vi "Path_Test_TankRobot_ScanIndex_CreateFile.vi"() -> ()   [LabVIEW 2018]
uses:
  Pathfinder-Lib/VIs/Waypoint.ctl
  <vilib>/Rock Robotics/WPI/DriverStation/WPI_DriverStationRobotMode2.ctl
  Pathfinder-Lib/VIs/Wheel_Ctrl_Path_Element.ctl
  Pathfinder-Lib/VIs/Wheel_Ctrl_Path.ctl
  Pathfinder-Lib/Pathfinder.lvlib
  Robot Global Data.vi
  <vilib>/Rock Robotics/SystemInterfaces/AI/FPGA_AIGyroChannel.ctl
  <vilib>/Rock Robotics/Network Tables/NT Write Number.vi
  <vilib>/Rock Robotics/WPI/Counter/WPI_CounterDigitalInputToDigitalSource.vi
  <vilib>/Rock Robotics/SystemInterfaces/DIO/FPGA_DIOChannel.ctl
  <vilib>/Rock Robotics/WPI/Encoder/WPI_EncoderType.ctl
  <vilib>/Rock Robotics/Network Tables/NT Write Numeric Array.vi
  <vilib>/addons/control/pid/NI_PID_pid.lvlib
  <vilib>/Rock Robotics/SystemInterfaces/DIO/FPGA_DIOPWMChannel.ctl
  <vilib>/Rock Robotics/WPI/SafetyOutput/WPI_SafetyOutputConfigMenu.ctl
  Secret_Control_Library_Protected/Secret_Control_Library_Protected.lvlib
  <vilib>/addons/control/pid/pid.llb/PID (DBL).vi
  <vilib>/Rock Robotics/WPI/Gyro/WPI_GyroAnalogOpen.vi
  <vilib>/Rock Robotics/WPI/RobotDrive/WPI_RobotDriveOpen2MotorWithTalon.vi
panel:
  out "Path \nSpeed > \nMax":bool
  in  "Stop\nProgram":bool
  out "Path Distance":dbl[](array[numeric]) format="%19.2f"
  out "Robot\nExecuting":bool
  in  "Execute\nPath":bool
  out "Ready to \nExecute":bool
  in  "Calculate\nPath":bool
  out "Heading Demand":dbl format="%18.2f"
  out "Gyro Comp":dbl format="%18.2f"
  out "Heading":dbl format="%18.2f"
  in  "Gyro Comp PID gains":T1={"proportional gain (Kc)"=0.065, "integral time (Ti, min)"=0.004, "derivative time (Td, min)"=0.0} {"derivative time (Td, min)" format="%.4f"; "integral time (Ti, min)" format="%.4f"; "proportional gain (Kc)" format="%.4f"}
  out "Path calculation error":errorcluster
  out "Distance":dbl[](array[numeric]) format="%19.2f"
  in  "Use Gyro\nCompensation":bool=TRUE
  out "Heading Error":dbl format="%14.2f"
  out "Distance Error":dbl[](array[numeric]) format="%14.2f"
  out "Robot Mode":T2
  in  "Tab Control":T3(tab)
  in  "max_velocity":dbl=70.0
  in  "max_acceleration":dbl=65.0
  in  "max_jerk":dbl=120.0
  in  "wheelbase_width":dbl=20.866
  in  "Real max\n speed":dbl=84.0
  out "Position":cluster{dbl[], dbl[]}[](graph)
  out "Path":T4(graph)
  out "Size":i32
  out "Robot Path Data":T5[](array[typedef]) {"D Time" format="%13.3f"; "Angle" format="%13.3f"; "R dist" format="%13.3f"; "L dist" format="%13.3f"; "R spd" format="%13.3f"; "L spd" format="%13.3f"; "T Time" format="%13.3f"}
  out "Wheel dmd":T6(graph)
  out "Gyro Cht":cluster{"GyroContinuous":dbl, "Angle":dbl}(graph)
  out "Err Chart":cluster{dbl, dbl, dbl}(graph)
  in  "CreateCmdList":bool
  in  "Command List File Name":path
  in  "Command List Path Comment":string
  in  "Starting Step":i32
  in  "Start Path CMD":i32=60
  in  "Cont Path CMD":i32=62
  in  "End Path CMD":i32=64
  in  "Include Step":bool
  in  "sample_count":i32=1000
  in  "Path Results\ndT":dbl=0.02 format="%7.3f"
  in  "?":T7[](array[typedef])=[{"x"=12.0, "y"=60.0, "angle"=0.0}, {"x"=132.0, "y"=125.0, "angle"=60.0}]
  # "PATH DEFINITION"
  # "ROBOT EXECUTION\n(disabled...)"
  # "SEC"
  # "Instructions:\nThis should run on a PC simulated robot on or a real robot that has the same motors and sensors.\n1) Enter robot data on Robot Data Tab\n2) Define your path definitions.\n3) Define the time increment.  0.020 is chosen since that matches the normal loop time.\n4) Press calculate path.  If a good path was calculated it will be displayed on the Tank Data tab, and the Ready to Execute will indicate execution can begin.\nThe path can be recalculated many times before selecting execute.\n5) Start the FRC driver station.\n6) Press the execute path button.  This will start the robot simulation, or start running on the roboRIO depending on which target is selected.\n7) On the driver station, select Autonomous Enabled mode to start path execution.\n8) When finished, the graph tabs can be reviwed.  (Usiing the chart tabs during operation breaks the simulation.\n9) When completely done press the Stop Program button to end the programs execution.\n\nNotes:\n- This program alters the left and right motor demands during execution to attempt to match the heading angle demand.  The \nsimulated robot has a lot of drive friction when turning that affects operation.  This example does not include encoder compensation.\nThis could be added.\n- The path generation logic doesn't account distribution of speed to the left and right wheels.  As a result the maximum speed can be exceeded.\nIf this happens, but Path Speed > Max light will light and Ready to Execute will not light.  Lower the maximum speed in the Robot Data tab\nand recalulate the path."
  # "ROBOT DATA"
  # "INCHES/SEC"
  # "INCHES/SEC"
  # "INCHES/SEC^2"
  # "?? INCHES/SEC^3"
  # "Simulated robot is 20.866"
  # "INCHES"
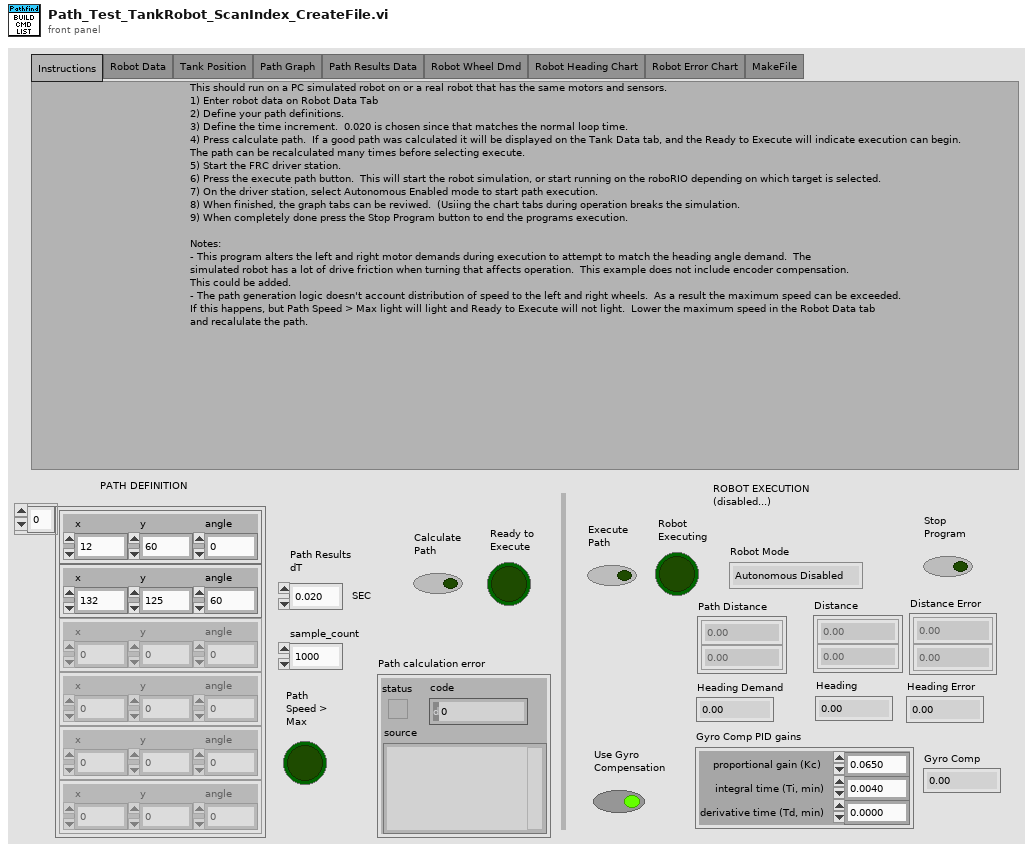
[diagram p1: front panel]
types:
  T1 = cluster{"proportional gain (Kc)":dbl, "integral time (Ti, min)":dbl, "derivative time (Td, min)":dbl}
  T2 = typedef "WPI_DriverStationRobotMode2.ctl" = enum16{"Autonomous Disabled", "Autonomous Enabled", "Teleop Disabled", "Teleop Enabled", "Disconnected", "Finish", "Test Disabled", "Test Enabled", "Emergency Stopped"}
  T3 = enum32{"Instructions", "Robot Data", "Tank Position", "Path Graph", "Path Results Data", "Robot Wheel Dmd", "Robot Heading Chart", "Robot Error Chart", "MakeFile"}
  T4 = cluster{"position":dbl, "velocity":dbl, "acceleration":dbl, "jerk":dbl, "heading":dbl}[]
  T5 = typedef "Pathfinder.lvlib/Wheel_Ctrl_Path_Element.ctl" = cluster{"T Time":dbl, "L spd":dbl, "R spd":dbl, "L dist":dbl, "R dist":dbl, "Angle":dbl, "D Time":dbl}
  T6 = cluster{"Output":dbl, "Output":dbl, "output":dbl}
  T7 = typedef "Pathfinder.lvlib/Waypoint.ctl" = cluster{"x":dbl, "y":dbl, "angle":dbl}
  T8 = typedef "Pathfinder.lvlib/Wheel_Ctrl_Path.ctl" = cluster{"Wheel_Ctrl_Elements":T5[], "NumberOfElements":u32, "DeltaMillseconds":i32}
  T9 = enum32{"Instructions", "Robot Data", "Tank Position", "Path Graph", "Path Results Data", "Robot Wheel Dmd", "Robot Heading Chart", "Robot Error Chart"}
  T10 = typedef "Pathfinder.lvlib/Segment.ctl" = cluster{"dt":dbl, "x":dbl, "y":dbl, "position":dbl, "velocity":dbl, "acceleration":dbl, "jerk":dbl, "heading":dbl}
  T11 = cluster{"position":dbl, "velocity":dbl, "acceleration":dbl, "jerk":dbl, "heading":dbl}
  T12 = typedef "WPI_SafetyOutputConfigMenu.ctl" = enum16{"Enable", "Disable"}
  T13 = typedef "WPI_EncoderType.ctl" = enum16{"1x", "2x", "4x"}
  T14 = typedef "FPGA_AIGyroChannel.ctl" = enum8{"AI 0", "AI 1", "Invalid"}
  T15 = typedef "FPGA_DIOPWMChannel.ctl" = enum8{"PWM 0", "PWM 1", "PWM 2", "PWM 3", "PWM 4", "PWM 5", "PWM 6", "PWM 7", "PWM 8", "PWM 9", "PWM MXP 0", "PWM MXP 1", "PWM MXP 2", "PWM MXP 3", "PWM MXP 4", "PWM MXP 5", "PWM MXP 6", "PWM MXP 7", "PWM MXP 8", "PWM MXP 9", "Invalid"}
  T16 = typedef "FPGA_DIOChannel.ctl" = enum8{"DIO 0", "DIO 1", "DIO 2", "DIO 3", "DIO 4", "DIO 5", "DIO 6", "DIO 7", "DIO 8", "DIO 9", "DIO MXP 0", "DIO MXP 1", "DIO MXP 2", "DIO MXP 3", "DIO MXP 4", "DIO MXP 5", "DIO MXP 6", "DIO MXP 7", "DIO MXP 8", "DIO MXP 9", "DIO MXP 10", "DIO MXP 11", "DIO MXP 12", "DIO MXP 13", "DIO MXP 14", "DIO MXP 15", "SPI Port CS1", "SPI Port CS2", "SPI Port CS3", "SPI Port MISO", "SPI Port MOSI", "Invalid"}
  T17 = typedef "WPI_RobotDriveDevRef.ctl" = cluster{"DevStatus":errorcluster, "Motors[]":T18[], "Square Inputs":bool, "Max Output":dbl}
  T18 = typedef "WPI_MotorControlDeviceRef.ctl" = cluster{"DeviceStatus":errorcluster, "Type":T19, "PWM":cluster{"PWM Channel":T15, "DeadBand":T20}, "CAN":cluster{"Device Number":u8, "SetOutput VI Ref":variant, "GetOutput VI Ref":variant, "Enable VI Ref":variant, "Disable VI Ref":variant, "Data":variant}, "Invert":bool, "DIO PWM":cluster{"PWM \"Enable\" Channel":T15, "DIOChannel":T16, "PWM Rate":dbl}}
  T19 = typedef "WPI_MotorControlType.ctl" = enum16{"PWM", "CAN", "DIO PWM"}
  T20 = typedef "WPI_PWMDeadband.ctl" = cluster{"Name":string, "maxPositivePwm":i32, "minPositivePwm":i32, "centerPwm":i32, "maxNegativePwm":i32, "minNegativePwm":i32, "angularRange":u16}
  T21 = typedef "WPI_DigitalInputDevRef.ctl" = cluster{"DevStatus":errorcluster, "DIO Channel":T16}
  T22 = typedef "FPGA_CounterEncoderSourceConvertionLVSourceType.ctl" = cluster{"DevStatus":errorcluster, "AnalogTriggerMode?":bool, "DigitalMode":cluster{"DIO Channel":T23}, "AnalogTriggerMode":cluster{"AnalogTriggerIndex":T24, "OutputType":T25}}
  T23 = typedef "FPGA_DIODigitalSourceChannel.ctl" = enum8{"DIO 0", "DIO 1", "DIO 2", "DIO 3", "DIO 4", "DIO 5", "DIO 6", "DIO 7", "DIO 8", "DIO 9", "DIO MXP 0", "DIO MXP 1", "DIO MXP 2", "DIO MXP 3", "DIO MXP 4", "DIO MXP 5", "DIO MXP 6", "DIO MXP 7", "DIO MXP 8", "DIO MXP 9", "DIO MXP 10", "DIO MXP 11", "DIO MXP 12", "DIO MXP 13", "DIO MXP 14", "DIO MXP 15", "SPI Port CS1", "SPI Port CS2", "SPI Port CS3", "SPI Port MISO", "SPI Port MOSI", "Disabled"}
  T24 = typedef "FPGA_AnalogTriggerIndex.ctl" = enum8{"Trig 0", "Trig 1", "Trig 2", "Trig 3", "Trig 4", "Trig 5", "Trig 6", "Trig 7", "Invalid"}
  T25 = typedef "FPGA_AnalogTriggerOutType.ctl" = enum16{"InWindow", "TriggerState", "Rising", "Falling"}
  T26 = typedef "WPI_EncoderDevRef.ctl" = cluster{"DevStatus":errorcluster, "EncoderIndex":T27, "CounterIndex":T28, "DistancePerCount":dbl, "Decoding Type":T13}
  T27 = typedef "FPGA_EncoderIdx.ctl" = enum8{"Enc 0", "Enc 1", "Enc 2", "Enc 3", "Enc 4", "Enc 5", "Enc 6", "Enc 7", "Invalid"}
  T28 = typedef "FPGA_CounterCtrSystemIndex.ctl" = enum8{"Ctr 0", "Ctr 1", "Ctr 2", "Ctr 3", "Ctr 4", "Ctr 5", "Ctr 6", "Ctr 7", "Invalid"}
  T29 = typedef "WPI_GyroDevRef.ctl" = cluster{"DevStatus":errorcluster, "Analog Channel":T30, "Gain (VoltsPerDegree/Second)":dbl, "Gyro Type":enum16{"Analog", "XRS450"}, "Handle":i32, "SPI Bus":T31, "Device Found":bool, "Sample Rate":dbl, "Calibrate On Open":bool, "Offset":dbl}
  T30 = typedef "FPGA_AIChannel.ctl" = enum8{"AI 0", "AI 1", "AI 2", "AI 3", "AI MXP 0", "AI MXP 1", "AI MXP 2", "AI MXP 3", "Invalid"}
  T31 = typedef "spi_bus.ctl" = enum16{"SPI On-Board, CS0", "SPI On-Board, CS1", "SPI On-Board, CS2", "SPI On-Board, CS3", "SPI MXP", "Invalid"}
  T32 = cluster{"GyroContinuous":dbl, "GyroContinuous":dbl}
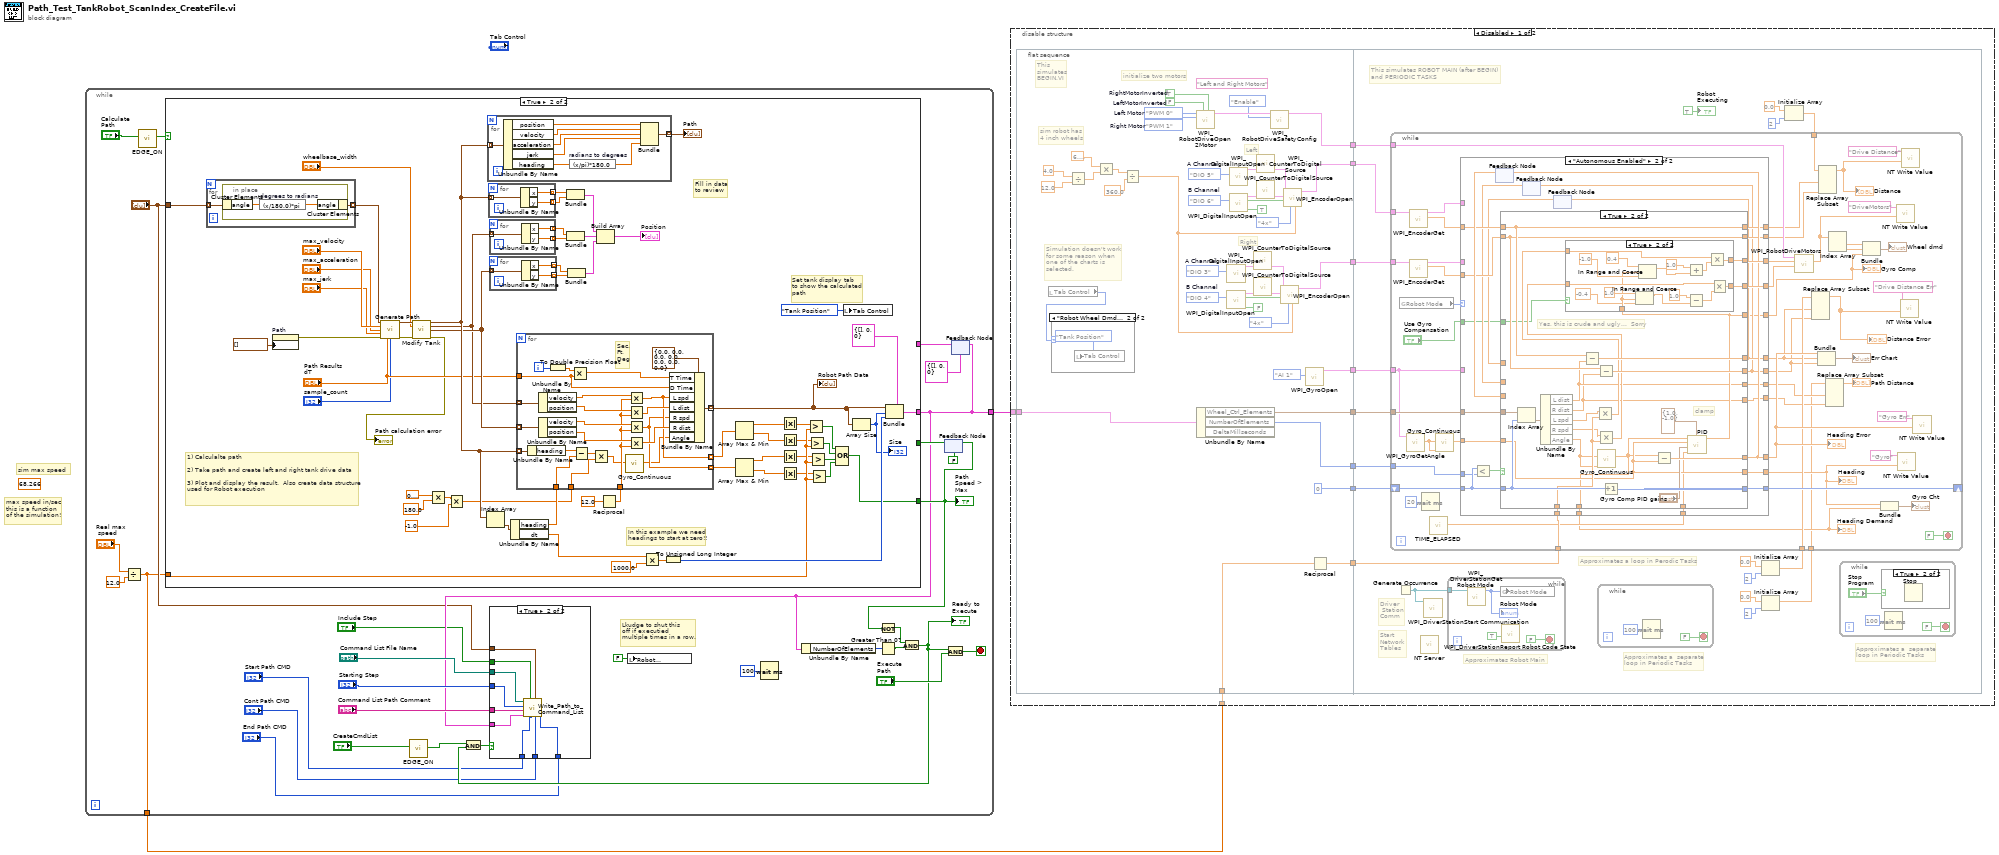
[diagram p0: block diagram]
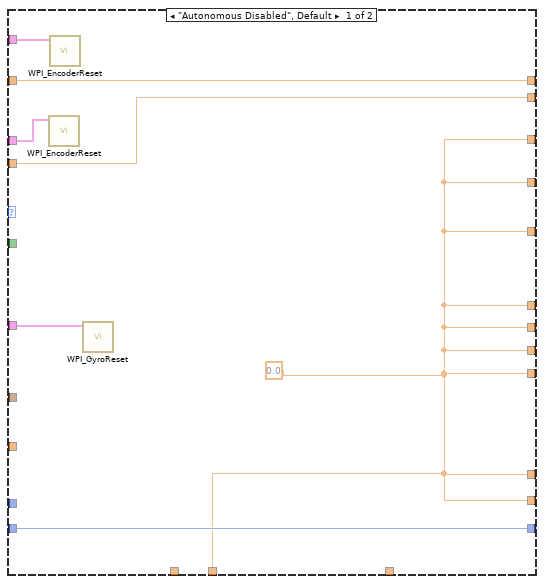
[diagram p4: hidden frame]
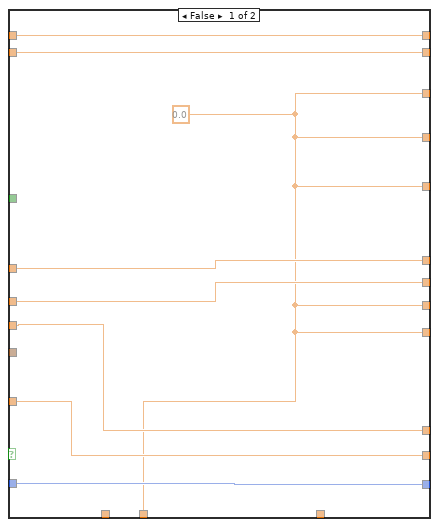
[diagram p5: hidden frame]
diagram:
  (unwired) 68.266 ("x")
  # "sim max speed"
  # "max speed in/sec\nthis is a function\nof the simulation!"
  n1 = while {
    tunnel: [w11] -> w2
    tunnel: [w3] -> w1
    stop <- w25 stop-if-true
    # "Lkudge to shut this\noff if executied\nmultiple times in a row."
    n2 = Divide(x="Real max\n speed", y=12.0) -> (x/y=w3:dbl)
    n3 = call "EDGE_ON.vi"("INPUT"="Calculate\nPath") -> ("EDGE ON"=w30:bool)  [unwired: 10 in]
    n4 = call "EDGE_ON.vi"("INPUT"="CreateCmdList") -> ("EDGE ON"=w13:bool)  [unwired: 10 in]
    n5 = local write "Robot\nExecuting"(FALSE ("Robot\nExecuting")) -> ()
    n6 = Wait (ms)(milliseconds to wait=u32 100) -> ()  [unwired: 1 out]
    n7 = feedback #1(FALSE) -> (w22:bool)
    n8 = feedback #2(T8 {"Wheel_Ctrl_Elements"=[], "NumberOfElements"=0, "DeltaMillseconds"=0} ("Wheel_Ctrl_Elements")) -> (w28:T8)
    n9 = case shown="True" w30 {
      tunnel: [w43 w65] -> w11
      tunnel: w28 -> [w43 _]
      tunnel: w3 -> [_ w63]
      tunnel: [w42 w54] -> w19
      tunnel: w22 -> [w42 _]
      tunnel: "?" -> [_ w44]
      frame False {
      }
      frame True {
        # "Set tank display tab\nto show the calculated\npath"
        # "Fill in data\nto review"
        # "1) Calculalte path\n\n2) Take path and create left and right tank drive data\n\n3) Plot and display the result.  Also create data structure\nused for Robot execution"
        # "In this example we need\nheadings to start at zero!!"
        n10 = for {
          tunnel: w44 -> [w130] mode=indexing
          tunnel: [w129] -> w91 mode=indexing
          n11 = in-place {
            n12 = in-place-cluster #3(w130) -> ("angle"=w132:dbl)
            n13 = expression code="(x/180.0)*pi" "degrees to radians"(w132) -> (w131:dbl)
            n14 = in-place-cluster #3("angle"=w131) -> (w129:T7)
          }
        }
        n15 = property on="Path" class="WFChart (strict)"("History Data"=T4 []) -> (error out=w92:errorcluster)  [unwired: 2 in, 1 out]
        n16 = call "Generate Path.vi"("path"=w91, "max_velocity"="max_velocity", "max_acceleration"="max_acceleration", "max_jerk"="max_jerk", "error in"=w92, "dt (.001)"="Path Results\ndT", "sample_count (100000)"="sample_count") -> ("Segments"=w93:T10[], "error out"=w80:errorcluster)  [unwired: 7 in]
        n17 = call "Modify Tank.vi"("Original"=w93, "wheelbase_width"="wheelbase_width", "error in"=w80) -> ("original"=w102:T10[], "left"=w98:T10[], "right"=w99:T10[], "error out"=→"Path calculation error":errorcluster)  [unwired: 9 in]
        n18 = Multiply(x=0.3183098861837907, y=180.0) -> (x*y=w101:dbl)
        n19 = Multiply(x=w101, y=-1.0) -> (x*y=w45:dbl)
        n20 = Index Array(array=w102) -> (element=w103:T10)  [unwired: 1 in]
        n21 = for {
          tunnel: w102 -> [w149] mode=indexing
          tunnel: [w143] -> w95 mode=indexing
          n22 = Unbundle By Name(w149) -> ("position"=w148:dbl, "velocity"=w147:dbl, "acceleration"=w146:dbl, "jerk"=w145:dbl, "heading"=w144:dbl)
          n23 = expression code="(x/pi)*180.0" "radians to degrees"(w144) -> (w142:dbl)
          n24 = Bundle("position"=w148, "velocity"=w147, "acceleration"=w146, "jerk"=w145, "heading"=w142) -> (w143:T11)  [unwired: 1 in]
        }
        "Path" <- w95
        n25 = for {
          tunnel: w102 -> [w135] mode=indexing
          tunnel: [w134] -> w88 mode=indexing
          tunnel: [w133] -> w89 mode=indexing
          n26 = Unbundle By Name(w135) -> ("x"=w134:dbl, "y"=w133:dbl)
        }
        n27 = for {
          tunnel: w98 -> [w141] mode=indexing
          tunnel: [w140] -> w82 mode=indexing
          tunnel: [w139] -> w83 mode=indexing
          n28 = Unbundle By Name(w141) -> ("x"=w140:dbl, "y"=w139:dbl)
        }
        n29 = for {
          tunnel: w99 -> [w138] mode=indexing
          tunnel: [w137] -> w84 mode=indexing
          tunnel: [w136] -> w85 mode=indexing
          n30 = Unbundle By Name(w138) -> ("x"=w137:dbl, "y"=w136:dbl)
        }
        n31 = Unbundle By Name(w103) -> ("heading"=w104:dbl, "dt"=w69:dbl)
        n32 = Bundle(w88, w89) -> (w90:cluster{dbl[], dbl[]})  [unwired: 1 in]
        n33 = Bundle(w82, w83) -> (w87:cluster{dbl[], dbl[]})  [unwired: 1 in]
        n34 = Bundle(w84, w85) -> (w86:cluster{dbl[], dbl[]})  [unwired: 1 in]
        n35 = Build Array(w90, w87, w86) -> (→"Position":cluster{dbl[], dbl[]}[])
        n36 = Reciprocal(x=12.0) -> (1/x=w97:dbl)
        n37 = for {
          tunnel: "Path Results\ndT" -> [w124]
          tunnel: [w127] -> w53 mode=indexing
          tunnel: w97 -> [w119]
          tunnel: w98 -> [w116] mode=indexing
          tunnel: w99 -> [w115] mode=indexing
          tunnel: w102 -> [w114] mode=indexing
          tunnel: w104 -> [w107]
          tunnel: [w110] -> w52 mode=indexing
          tunnel: [w109] -> w51 mode=indexing
          tunnel: w45 -> [w108]
          i -> [w126]
          # "Sec,\nFt,\nDeg"
          n38 = Unbundle By Name(w114) -> ("heading"=w112:dbl)
          n39 = Unbundle By Name(w116) -> ("velocity"=w123:dbl, "position"=w122:dbl)
          n40 = Unbundle By Name(w115) -> ("velocity"=w121:dbl, "position"=w120:dbl)
          n41 = To Double Precision Float(number=w126) -> (double precision float=w128:dbl)
          n42 = Multiply(x=w128, y=w124) -> (x*y=w125:dbl)
          n43 = Subtract(x=w112, y=w107) -> (x-y=w113:dbl)
          n44 = Multiply(x=w113, y=w108) -> (x*y=w106:dbl)
          n45 = call "Gyro_Continuous.vi"("GyroInput"=w106) -> ("GyroContinuous"=w105:dbl)  [unwired: 10 in]
          n46 = Multiply(x=w123, y=w119) -> (x*y=w110:dbl)
          n47 = Multiply(x=w122, y=w119) -> (x*y=w118:dbl)
          n48 = Multiply(x=w121, y=w119) -> (x*y=w109:dbl)
          n49 = Multiply(x=w120, y=w119) -> (x*y=w117:dbl)
          n50 = Bundle By Name(cluster=T5 {"T Time"=0.0, "L spd"=0.0, "R spd"=0.0, "L dist"=0.0, "R dist"=0.0, "Angle"=0.0, "D Time"=0.0} ("Wheel dmd"), "T Time"=w125, "D Time"=w124, "L spd"=w110, "L dist"=w118, "R spd"=w109, "R dist"=w117, "Angle"=w105) -> (w127:T5)
        }
        "Robot Path Data" <- w53
        n51 = Multiply(x=w69, y=1000.0) -> (x*y=w67:dbl)
        n52 = To Unsigned Long Integer(number=w67) -> (unsigned 32bit integer=w66:u32)
        n53 = Array Max & Min(array=w52) -> (max value=w50:dbl, min value=w49:dbl)  [unwired: 2 out]
        n54 = Array Max & Min(array=w51) -> (max value=w48:dbl, min value=w47:dbl)  [unwired: 2 out]
        n55 = Absolute Value(x=w50) -> (abs(x)=w62:dbl)
        n56 = Absolute Value(x=w49) -> (abs(x)=w61:dbl)
        n57 = Absolute Value(x=w48) -> (abs(x)=w60:dbl)
        n58 = Absolute Value(x=w47) -> (abs(x)=w59:dbl)
        n59 = Greater?(x=w62, y=w63) -> (0:w58:bool)
        n60 = Greater?(x=w61, y=w63) -> (0:w57:bool)
        n61 = Greater?(x=w60, y=w63) -> (0:w56:bool)
        n62 = Greater?(x=w59, y=w63) -> (0:w55:bool)
        n63 = Compound Arithmetic op=OR(w58, w57, w56, w55) -> (w54:bool)
        n64 = local write "Tab Control"(T9."Tank Position" ("Tab Control")) -> ()
        n65 = Array Size(array=w53) -> (size(s)=w64:i32)
        "Size" <- w64
        n66 = Bundle(cluster=T8 {"Wheel_Ctrl_Elements"=[], "NumberOfElements"=0, "DeltaMillseconds"=0} ("Wheel_Ctrl_Elements"), "Wheel_Ctrl_Elements"=w53, "NumberOfElements"=w64, "DeltaMillseconds"=w66) -> (w65:T8)
      }
    }
    "Path \nSpeed > \nMax" <- w19
    n67 = Unbundle By Name(w11) -> ("NumberOfElements"=w27:u32)
    n68 = Not(x=w19) -> (.not. x?=w20:bool)
    n69 = Greater Than 0?(x=w27) -> (x > 0?=w21:bool)
    n70 = And(x=w20, y=w21) -> (x .and. y?=w12:bool)
    "Ready to \nExecute" <- w12
    n71 = And(x=w13, y=w12) -> (x .and. y?=w14:bool)
    n72 = case shown="True" w14 {
      tunnel: "Command List File Name" -> [_ w41]
      tunnel: "Starting Step" -> [_ w40]
      tunnel: "Command List Path Comment" -> [_ w39]
      tunnel: w11 -> [_ w38]
      tunnel: "End Path CMD" -> [_ w37]
      tunnel: "Cont Path CMD" -> [_ w36]
      tunnel: "Start Path CMD" -> [_ w35]
      tunnel: "Include Step" -> [_ w34]
      tunnel: "?" -> [_ w33]
      frame False {
      }
      frame True {
        n73 = call "Write_Path_to_Command_List.vi"("LastCmdNumb"=w37, "CmdNumb"=w36, "WayPoints"=w33, "FirstCmdNumb"=w35, "Include Step"=w34, "Wheel_Ctrl_Elements"=w38, "Comment"=w39, "starting step"=w40, "Cmd List File"=w41) -> ()  [unwired: 3 in]
      }
    }
    n74 = feedback-in #1(w19) -> ()
    n75 = And(x=w12, y="Execute\nPath") -> (x .and. y?=w25:bool)
    n76 = feedback-in #2(w11) -> ()
  }
  n77 = disable-structure shown="Disabled" {
    disable-tunnel: w1 -> [w151 _]
    disable-tunnel: w2 -> [w150 _]
    frame Disabled {
      n78 = flat-sequence {
        tunnel: w150 -> [w166]
        tunnel: [w169] -> w159
        tunnel: [w199] -> w158
        tunnel: [w167] -> w157
        tunnel: [w168] -> w156
        tunnel: [w165] -> w155
        tunnel: [w164] -> w154
        tunnel: [w163] -> w153
        tunnel: w151 -> [w162]
        tunnel: [0] -> w152
        tunnel: w159 -> [w218]
        tunnel: w158 -> [w217]
        tunnel: w157 -> [w216]
        tunnel: w156 -> [w209]
        tunnel: w155 -> [w219]
        tunnel: w154 -> [w208]
        tunnel: w153 -> [w203]
        tunnel: w152 -> [w202]
        frame #0 {
          w183 = FPGA_DIOPWMChannel."PWM 1"  # Right Motor
          w182 = FPGA_DIOPWMChannel."PWM 0"  # Left Motor
          (unwired) "Left and Right Motors" ("refnum name")
          w184 = FALSE  # LeftMotorInverted
          w185 = TRUE  # RightMotorInverted
          w177 = FPGA_DIOChannel."DIO 4"  # B Channel
          w176 = FPGA_DIOChannel."DIO 3"  # A Channel
          w173 = FPGA_DIOChannel."DIO 6"  # B Channel
          w172 = FPGA_DIOChannel."DIO 5"  # A Channel
          # "Simulation doesn't work\nfor some reason when\none of the charts is\nselected."
          # "This \nsimulates\nBEGIN.VI"
          # "sim robot has\n4 inch wheels"
          # "initialize two motors"
          # "Right"
          # "Left"
          n79 = local read "Tab Control"() -> (w160:T3)
          n80 = case shown="\"Robot Wheel Dmd\"..\"Robot Error Chart\"" w160 {
            frame Default {
            }
            frame "Robot Wheel Dmd".."Robot Error Chart" {
              n81 = local write "Tab Control"(T9."Tank Position" ("Tab Control")) -> ()
            }
          }
          n82 = Divide(x=4.0, y=12.0) -> (x/y=w195:dbl)
          n83 = Multiply(x=6.283185307179586, y=w195) -> (x*y=w196:dbl)
          n84 = Divide(x=w196, y=360.0) -> (x/y=w197:dbl)
          n85 = call-poly <vilib>:"WPI_RobotDriveOpen2Motor.vi"("Right Motor Inverted"=w185, "Left Motor Inverted"=w184, "Right Motor"=w183, "Left Motor"=w182) -> ("RobotDriveDevRef"=w198:T17)  [unwired: 1 in, 6 out]
          n86 = Unbundle By Name(w166) -> ("Wheel_Ctrl_Elements"=w165:T5[], "NumberOfElements"=w164:u32)  [unwired: 1 out]
          n87 = call <vilib>:"WPI_DigitalInputOpen.vi"("DIO Channel"=w176) -> ("DigitalInputDevRef"=w193:T21)  [unwired: 1 in, 9 out]
          n88 = call <vilib>:"WPI_DigitalInputOpen.vi"("DIO Channel"=w177) -> ("DigitalInputDevRef"=w192:T21)  [unwired: 1 in, 9 out]
          n89 = call <vilib>:"WPI_DigitalInputOpen.vi"("DIO Channel"=w172) -> ("DigitalInputDevRef"=w189:T21)  [unwired: 1 in, 9 out]
          n90 = call <vilib>:"WPI_DigitalInputOpen.vi"("DIO Channel"=w173) -> ("DigitalInputDevRef"=w188:T21)  [unwired: 1 in, 9 out]
          n91 = call-poly <vilib>:"WPI_CounterToDigitalSource.vi"("DigitalInputDevRef"=w193) -> ("Digital Source"=w194:T22)  [unwired: 6 out]
          n92 = call-poly <vilib>:"WPI_CounterToDigitalSource.vi"("DigitalInputDevRef"=w192) -> ("Digital Source"=w191:T22)  [unwired: 6 out]
          n93 = call-poly <vilib>:"WPI_CounterToDigitalSource.vi"("DigitalInputDevRef"=w189) -> ("Digital Source"=w190:T22)  [unwired: 6 out]
          n94 = call-poly <vilib>:"WPI_CounterToDigitalSource.vi"("DigitalInputDevRef"=w188) -> ("Digital Source"=w187:T22)  [unwired: 6 out]
          n95 = call <vilib>:"WPI_RobotDriveSafetyConfig.vi"("mode"=WPI_SafetyOutputConfigMenu."Enable", "RobotDriveDevRef"=w198) -> ("RobotDriveDevRef"=w169:T17)  [unwired: 8 in, 1 out]
          n96 = call <vilib>:"WPI_EncoderOpen.vi"("DistancePerCount"=w197, "Decoding Type"=WPI_EncoderType."4x", "Invert Direction (False)"=FALSE, "BSource"=w191, "ASource"=w194) -> ("EncoderDevRef"=w168:T26)  [unwired: 3 in, 3 out]
          n97 = call <vilib>:"WPI_EncoderOpen.vi"("DistancePerCount"=w197, "Decoding Type"=WPI_EncoderType."4x", "Invert Direction (False)"=TRUE, "BSource"=w187, "ASource"=w190) -> ("EncoderDevRef"=w167:T26)  [unwired: 3 in, 3 out]
          n98 = call-poly <vilib>:"WPI_GyroOpen.vi"("Analog Channel"=FPGA_AIGyroChannel."AI 1") -> ("GyroDevRef"=w199:T29)  [unwired: 8 in, 2 out]
          n99 = Reciprocal(x=w162) -> (1/x=w163:dbl)
        }
        frame #1 {
          # "Approximates a  separate\nloop in Periodic Tasks"
          # "This simulates ROBOT MAIN (after BEGIN)\nand PERIODIC TASKS"
          # "Approximates a loop in Perodic Tasks"
          # "Approximates a  separate\nloop in Periodic Tasks"
          # "Approximates Robot Main"
          # "Start\nNetwork\nTables"
          # "Driver\n Station\nComm"
          n100 = Generate Occurrence() -> (w220:refnum<k4>)
          n101 = call <vilib>:"NT Server.vi"() -> ()  [unwired: 12 in]
          n102 = call <vilib>:"WPI_DriverStationStart Communication.vi"("occurrence"=w220) -> ()  [unwired: 11 in]
          n103 = while {
            tunnel: w220 -> [w362]
            stop <- FALSE stop-if-true
            n104 = call <vilib>:"WPI_DriverStationGet Robot Mode.vi"("DS Occurrence"=w362) -> ("Robot Mode"=w359:T2)  [unwired: 1 in, 9 out]
            "Robot Mode" <- w359
            n105 = global write "Robot Global Data.vi" "Robot Mode"(w359) -> ()
            n106 = call <vilib>:"WPI_DriverStationReport Robot Code State.vi"("TeleOp"=TRUE ("Autonomous")) -> ()  [unwired: 10 in, 1 out]
          }
          n107 = while {
            stop <- FALSE stop-if-true
            n108 = Wait (ms)(milliseconds to wait=u32 100) -> ()  [unwired: 1 out]
          }
          n109 = Initialize Array(0.0, 2 ("dimension size")) -> (w210:dbl[])
          n110 = Initialize Array(0.0, 2 ("dimension size")) -> (w204:dbl[])
          n111 = Initialize Array(0.0, 2 ("dimension size")) -> (w213:dbl[])
          n112 = while {
            tunnel: w219 -> [w265]
            tunnel: w218 -> [w270]
            shift-right: [w266] -> _
            shift-left: w202 -> [w267]
            tunnel: w217 -> [w262]
            tunnel: w216 -> [w260]
            tunnel: w203 -> [w254]
            tunnel: w213 -> [w250]
            tunnel: w210 -> [w246]
            tunnel: w209 -> [w230]
            tunnel: w208 -> [w229]
            tunnel: w204 -> [w225]
            stop <- FALSE stop-if-true
            n113 = global read "Robot Global Data.vi" "Robot Mode"() -> (w271:T2)
            n114 = call <vilib>:"WPI_GyroGetAngle.vi"("GyroDevRef"=w262) -> ("Angle"=w236:dbl)  [unwired: 7 in, 3 out]
            n115 = call <vilib>:"WPI_EncoderGet.vi"("EncoderDevRef"=w260) -> ("Distance"=w257:dbl, "EncoderDevRef"=w231:T26)  [unwired: 5 in, 4 out]
            n116 = call <vilib>:"WPI_EncoderGet.vi"("EncoderDevRef"=w230) -> ("Distance"=w256:dbl, "EncoderDevRef"=w259:T26)  [unwired: 5 in, 4 out]
            n117 = Wait (ms)(milliseconds to wait=u32 20) -> ()  [unwired: 1 out]
            n118 = call "TIME_ELAPSED.vi"() -> ("Elapsed Sec"=w235:dbl)  [unwired: 11 in]
            n119 = call "Gyro_Continuous.vi"("GyroInitial"=w236, "GyroInput"=w236) -> ("GyroContinuous"=w242:dbl)  [unwired: 9 in]
            n120 = case shown="\"Autonomous Enabled\"" w271 {
              tunnel: [w273 w302] -> w269
              tunnel: [w273 w303] -> w268
              tunnel: w267 -> [w279 w305]
              tunnel: [w279 w304] -> w266
              tunnel: w265 -> [_ w301]
              tunnel: w254 -> [_ w299]
              tunnel: w262 -> [w278 _]
              tunnel: w242 -> [_ w298]
              tunnel: [w273 w297] -> w233
              tunnel: [w273 w296] -> w252
              tunnel: w259 -> [w277 _]
              tunnel: w257 -> [w276 w294]
              tunnel: w256 -> [w275 w293]
              tunnel: [w276 w292] -> w249
              tunnel: [w275 w291] -> w248
              tunnel: [w273 w287] -> w243
              tunnel: [w273 w288] -> w244
              tunnel: "Use Gyro\nCompensation" -> [_ w286]
              tunnel: [w273 w285] -> w238
              tunnel: w235 -> [_ w284]
              tunnel: [w273 w283] -> w232
              tunnel: w231 -> [w274 _]
              tunnel: w229 -> [_ w282]
              tunnel: [w273 w281] -> w227
              tunnel: [w273 w280] -> w226
              frame "Autonomous Disabled", Default {
                w273 = 0.0
                n121 = call <vilib>:"WPI_EncoderReset.vi"("EncoderDevRef"=w277) -> ()  [unwired: 9 in, 2 out]
                n122 = call <vilib>:"WPI_EncoderReset.vi"("EncoderDevRef"=w274) -> ()  [unwired: 9 in, 2 out]
                n123 = call <vilib>:"WPI_GyroReset.vi"("GyroDevRef"=w278) -> ()  [unwired: 9 in, 2 out]
              }
              frame "Autonomous Enabled" {
                n124 = Less?(x=w305, y=w282) -> (x < y?=w300:bool)
                n125 = feedback #4() -> (w295:dbl)  [unwired: 1 in]
                n126 = feedback #5() -> (w289:dbl)  [unwired: 1 in]
                n127 = feedback #6() -> (w290:dbl)  [unwired: 1 in]
                n128 = case shown="True" w300 {
                  tunnel: w305 -> [w313 w338]
                  tunnel: [w313 w339] -> w304
                  tunnel: [w306 w336] -> w303
                  tunnel: [w306 w335] -> w302
                  tunnel: w301 -> [_ w319]
                  tunnel: w299 -> [_ w337]
                  tunnel: w298 -> [w312 w323]
                  tunnel: [w312 w323] -> w297
                  tunnel: [w311 w327] -> w296
                  tunnel: w295 -> [w311 _]
                  tunnel: w294 -> [w309 w334]
                  tunnel: [w309 w334] -> w292
                  tunnel: w293 -> [w310 w333]
                  tunnel: [w310 w333] -> w291
                  tunnel: w290 -> [w308 _]
                  tunnel: w289 -> [w307 _]
                  tunnel: [w307 w332] -> w287
                  tunnel: [w308 w331] -> w288
                  tunnel: w286 -> [_ w328]
                  tunnel: [w306 w324] -> w285
                  tunnel: w284 -> [_ w322]
                  tunnel: [w306 w321] -> w283
                  tunnel: [w306 w315] -> w281
                  tunnel: [w306 w314] -> w280
                  frame False {
                    w306 = 0.0
                  }
                  frame True {
                    # "Yes, this is crude and ugly...  Sorry"
                    # "clamp"
                    n129 = Index Array(array=w319, index=w338) -> (element=w317:T5)
                    n130 = Unbundle By Name(w317) -> ("L dist"=w315:dbl, "R dist"=w314:dbl, "L spd"=w320:dbl, "R spd"=w316:dbl, "Angle"=w318:dbl)
                    n131 = Subtract(x=w334, y=w315) -> (x-y=w331:dbl)
                    n132 = Multiply(x=w320, y=w337) -> (x*y=w330:dbl)
                    n133 = Subtract(x=w333, y=w314) -> (x-y=w332:dbl)
                    n134 = Multiply(x=w316, y=w337) -> (x*y=w329:dbl)
                    n135 = call "Gyro_Continuous.vi"("GyroInitial"=w318, "GyroInput"=w318) -> ("GyroContinuous"=w321:dbl)  [unwired: 9 in]
                    n136 = Increment(x=w338) -> (x+1=w339:i32)
                    n137 = Subtract(x=w321, y=w323) -> (x-y=w327:dbl)
                    n138 = call-poly <vilib>:"PID.vi"("output range"=cluster{"output high":dbl, "output low":dbl} {"output high"=1.0, "output low"=-1.0}, "dt (s)"=w322, "PID gains"="Gyro Comp PID gains", "process variable"=w323, "setpoint"=w321) -> ("output"=w324:dbl)  [unwired: 5 in, 1 out]
                    n139 = case shown="True" w328 {
                      tunnel: [w340 w352] -> w336
                      tunnel: w330 -> [w341 w351]
                      tunnel: [w341 w350] -> w335
                      tunnel: w329 -> [w340 w349]
                      tunnel: w324 -> [_ w343]
                      frame False {
                      }
                      frame True {
                        n140 = In Range and Coerce(upper limit=1.0, x=w343, lower limit=-0.4 ("x")) -> (coerced(x)=w345:dbl)  [unwired: 1 out]
                        n141 = In Range and Coerce(upper limit=0.4, x=w343, lower limit=-1.0 ("x")) -> (coerced(x)=w346:dbl)  [unwired: 1 out]
                        n142 = Add(x=1.0, y=w346) -> (x+y=w355:dbl)
                        n143 = Subtract(x=1.0, y=w345) -> (x-y=w353:dbl)
                        n144 = Multiply(x=w351, y=w355) -> (x*y=w350:dbl)
                        n145 = Multiply(x=w349, y=w353) -> (x*y=w352:dbl)
                      }
                    }
                  }
                }
                n146 = feedback-in #4(w296) -> ()
                n147 = feedback-in #5(w287) -> ()
                n148 = feedback-in #6(w288) -> ()
              }
            }
            "Heading Error" <- w252
            "Heading" <- w233
            "Gyro Comp" <- w238
            "Heading Demand" <- w232
            n149 = call <vilib>:"WPI_RobotDriveMotors.vi"("RightSpeed"=w268, "LeftSpeed"=w269, "RobotDriveDevRef"=w270) -> ("Motor Values"=w241:dbl[])  [unwired: 6 in, 2 out]
            n150 = Replace Array Subset(array=w246, new element #1=w244, new element #2=w243) -> (w245:dbl[])  [unwired: 2 in]
            "Distance Error" <- w245
            n151 = Bundle(w252, w244, w243) -> (→"Err Chart":cluster{dbl, dbl, dbl})  [unwired: 1 in]
            n152 = Replace Array Subset(array=w250, new element #1=w249, new element #2=w248) -> (w247:dbl[])  [unwired: 2 in]
            "Distance" <- w247
            n153 = Replace Array Subset(array=w225, new element #1=w227, new element #2=w226) -> (→"Path Distance":dbl[])  [unwired: 2 in]
            n154 = Index Array(array=w241) -> (element #1=w239:dbl, element #2=w240:dbl)  [unwired: 2 in]
            n155 = Bundle("Output"=w239, "Output"=w240, "output"=w238) -> (→"Wheel dmd":T6)  [unwired: 1 in]
            n156 = Bundle("GyroContinuous"=w233, "GyroContinuous"=w232) -> (→"Gyro Cht":T32)  [unwired: 1 in]
            n157 = call-poly <vilib>:"NT Write Value.vi"("Numeric Array"=w241, "Name"="DriveMotors") -> ()  [unwired: 9 in, 1 out]
            n158 = call-poly <vilib>:"NT Write Value.vi"("Numeric"=w233, "Name"="Gyro") -> ()  [unwired: 9 in, 1 out]
            n159 = call-poly <vilib>:"NT Write Value.vi"("Numeric Array"=w245, "Name"="Drive Distance Err") -> ()  [unwired: 9 in, 1 out]
            n160 = call-poly <vilib>:"NT Write Value.vi"("Numeric Array"=w247, "Name"="Drive Distance") -> ()  [unwired: 9 in, 1 out]
            n161 = call-poly <vilib>:"NT Write Value.vi"("Numeric"=w252, "Name"="Gyro Err") -> ()  [unwired: 9 in, 1 out]
          }
          n162 = while {
            stop <- FALSE stop-if-true
            n163 = case shown="True" "Stop\nProgram" {
              frame False {
              }
              frame True {
                n164 = Stop() -> ()  [unwired: 1 in]
              }
            }
            n165 = Wait (ms)(milliseconds to wait=u32 100) -> ()  [unwired: 1 out]
          }
          "Robot\nExecuting" <- TRUE ("Robot\nExecuting")
        }
      }
    }
    frame Enabled {
    }
  }
